vi "XNETDB.Add.vi"(8 "error in (no error)":errorcluster, 11 "Databases Section Ref":T1 format="%.0x") -> (0 "error out":errorcluster)   [LabVIEW 2019, in "Diagnostics Addon Shared.lvlib"]
uses:
  Diagnostics Addon Shared.lvlib
  <vilib>/NI VeriStand/Custom Device API/Custom Device Item Ref.ctl
  NationalInstruments.VeriStand.Internal
  Constants.vi
  <vilib>/NI/NI VeriStand Advanced SysDef API/_SubVIs/SysDef.Property.Set.String.vi
  <vilib>/NI/NI VeriStand Advanced SysDef API/SysDef API/Advanced System Definition.lvlib
  <vilib>/NI VeriStand/Custom Device API/Custom Device API.lvlib
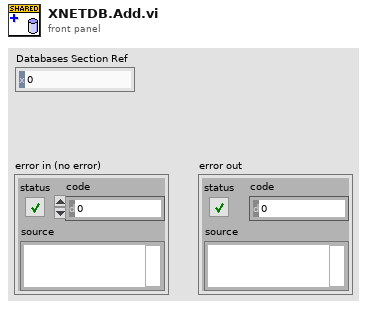
[diagram p1: front panel]
types:
  T1 = typedef "Custom Device API.lvlib/Custom Device Item Ref.ctl" = u64
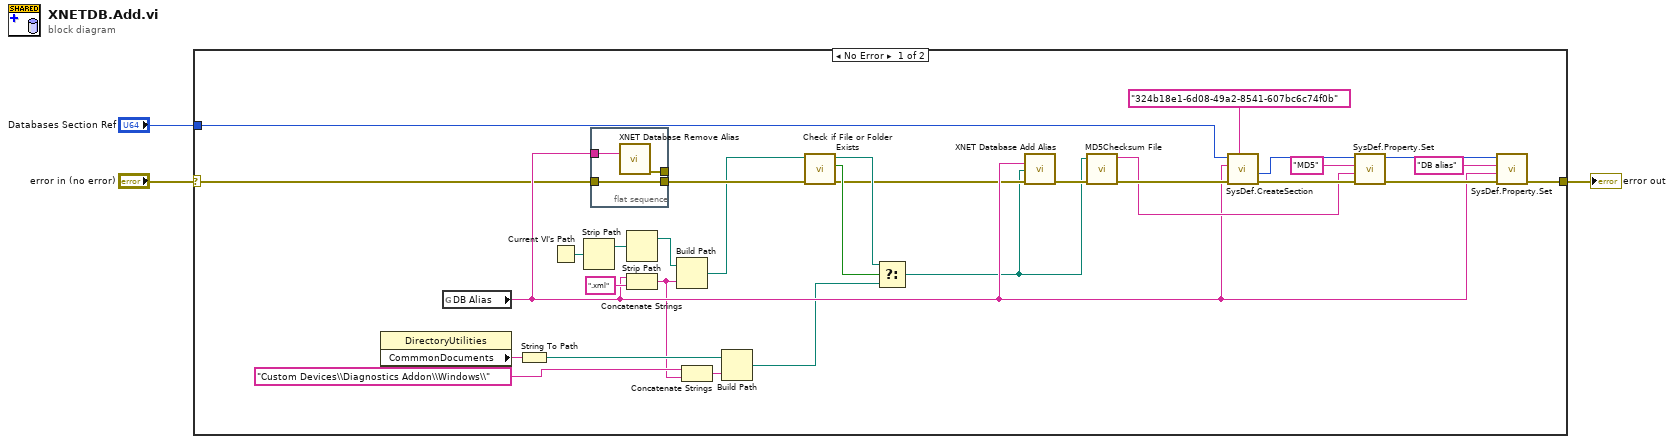
[diagram p0: block diagram]
diagram:
  n1 = case shown="No Error" "error in (no error)" {
    selector: "error in (no error)" -> [w4 w37]
    tunnel: "Databases Section Ref" -> [w33 _]
    tunnel: [w32 w37] -> w2
    frame No Error {
      n2 = property class="DirectoryUtilities"() -> ("CommmonDocuments"=w16:string)  [unwired: 2 in, 2 out]
      n3 = global read "Constants.vi" "DB Alias"() -> (w17:string)
      n4 = String To Path(string=w16) -> (path=w15:path)
      n5 = Current VI's Path() -> (path=w29:path)
      n6 = Strip Path(path=w29) -> (stripped path=w31:path)  [unwired: 1 out]
      n7 = flat-sequence {
        tunnel: [w36] -> w7
        tunnel: w4 -> [w36]
        tunnel: [w35] -> _
        tunnel: w17 -> [w34]
        frame #0 {
          n8 = call <vilib>:"XNET Database Remove Alias.vi"("alias"=w34) -> ("error out"=w35:errorcluster)  [unwired: 14 in]
        }
      }
      n9 = Strip Path(path=w31) -> (stripped path=w28:path)  [unwired: 1 out]
      n10 = Concatenate Strings(w17, ".xml" ("string")) -> (w12:string)
      n11 = Build Path(base path=w28, name or relative path=w12) -> (appended path=w6:path)
      n12 = Concatenate Strings("Custom Devices\\Diagnostics Addon\\Windows\\" ("name or relative path"), w12) -> (w13:string)
      n13 = Build Path(base path=w15, name or relative path=w13) -> (appended path=w9:path)
      n14 = call <vilib>:"Check if File or Folder Exists.vi"("error in (no error)"=w7, "path"=w6) -> ("error out"=w8:errorcluster, "file or folder exists?"=w11:bool, "dup path"=w10:path)  [unwired: 7 in]
      n15 = Select(t=w10, s=w11, f=w9) -> (s? t:f=w5:path)
      n16 = call <vilib>:"XNET Database Add Alias.vi"("alias"=w17, "filepath"=w5, "error in (no error)"=w8) -> ("error out"=w27:errorcluster)  [unwired: 12 in]
      n17 = call <vilib>:"MD5Checksum File.vi"("error in (no error)"=w27, "Path"=w5) -> ("error out"=w19:errorcluster, "MD5 message-digest"=w18:string)  [unwired: 8 in]
      n18 = call <vilib>:"SysDef.CreateSection.vi"("GUID"="324b18e1-6d08-49a2-8541-607bc6c74f0b" ("GUID (Default Section)"), "error in (no error)"=w19, "Name"=w17, "nodeID"=w33) -> ("error out"=w25:errorcluster, "New NodeID"=w26:u64)  [unwired: 4 in, 2 out]
      n19 = call-poly <vilib>:"SysDef.Property.Set.vi"("error in (no error)"=w25, "Value"=w18, "Property Name"="MD5", "nodeID"=w26) -> ("error out"=w24:errorcluster, "nodeID out"=w23:u64)  [unwired: 6 in]
      n20 = call-poly <vilib>:"SysDef.Property.Set.vi"("error in (no error)"=w24, "Value"=w17, "Property Name"="DB alias", "nodeID"=w23) -> ("error out"=w32:errorcluster)  [unwired: 6 in, 1 out]
    }
    frame Error {
    }
  }
  "error out" <- w2
